vi "Build Description String.vi"(8 "error in (no error)":errorcluster, 11 "Timing Action in":refnum<class "Timing Action.lvclass">) -> (0 "error out":errorcluster, 2 "Description":string, 3 "Timing Action out":refnum<class "Timing Action.lvclass">)   [LabVIEW 2020, in "MacroAssert.lvlib" / "Timing Action.lvclass"]
doc: "Builds a string to describe what <B>Step</B> does."
uses:
  Timing Action.lvclass
  Action Step/Action Step.lvclass
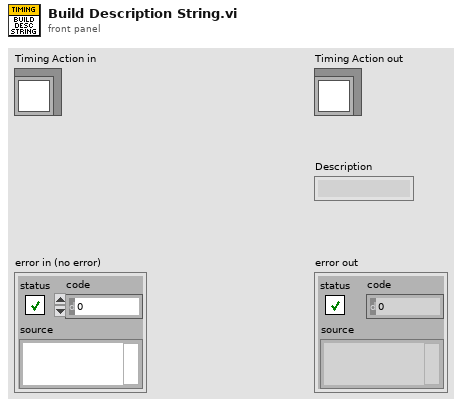
[diagram p1: front panel]
types:
  T1 = typedef "MacroAssert.lvlib/Timing Action.lvclass/Timing Action Type.ctl" = enum16{"Wait", "Wait Until"}
  T2 = typedef "MacroAssert.lvlib/Timing Action.lvclass/Time Unit.ctl" = enum16{"milliseconds", "seconds", "minutes"}
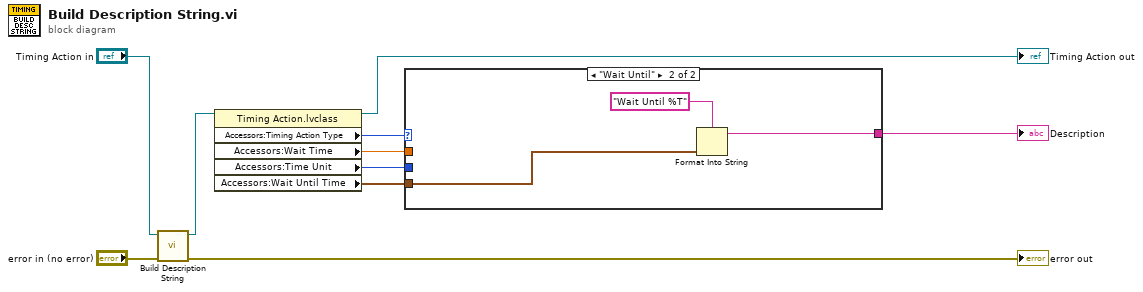
[diagram p0: block diagram]
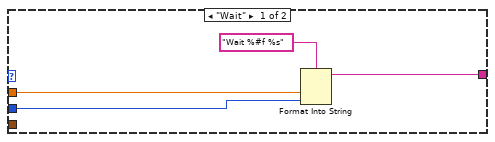
[diagram p2: hidden frame]
diagram:
  n1 = call-parent "Build Description String.vi"("error in (no error)"="error in (no error)", "Action Step in"="Timing Action in") -> ("error out"=→"error out":errorcluster, "Action Step out"=w9:refnum<class "Timing Action.lvclass">)  [unwired: 7 in, 1 out]
  n2 = property class="Timing Action.lvclass"(reference=w9) -> (reference out=→"Timing Action out":refnum<class "Timing Action.lvclass">, "Accessors:Timing Action Type"=w5:T1, "Accessors:Wait Time"=w4:dbl, "Accessors:Time Unit"=w3:T2, "Accessors:Wait Until Time"=w2:timestamp)  [unwired: 1 in, 1 out]
  n3 = case shown="\"Wait Until\"" w5 {
    tunnel: w4 -> [w13 _]
    tunnel: w3 -> [w12 _]
    tunnel: w2 -> [_ w15]
    tunnel: [w11 w16] -> w1
    frame "Wait" {
      n4 = Format Into String(format string="Wait %#f %s", w13, w12) -> (resulting string=w11:string)  [unwired: 2 in, 1 out]
    }
    frame "Wait Until" {
      n5 = Format Into String(format string="Wait Until %T", w15) -> (resulting string=w16:string)  [unwired: 2 in, 1 out]
    }
  }
  "Description" <- w1
